vi "Channel Mng Performance Test.vi"() -> ()   [LabVIEW 2021]
uses:
  <vilib>/Platform/TimedLoop/XDataNode/XDataNode.xnode
  <vilib>/Platform/TimedLoop/XDataNode/nitl_modes.ctl
  <vilib>/Platform/TimedLoop/XDataNode/XDNodeRunTimeDep.lvlib
  <vilib>/Platform/TimedLoop/XDataNode/wakeup.ctl
  <vilib>/Platform/TimedLoop/XDataNode/timing_clust.ctl
  7d13c5b7-0b44-4ab4-8a6c-0bcd63b70b59.vi
  6a1b8880-d4c2-444f-a4b2-811244e6db06.vi
  <vilib>/CIFChannels/CIFChannelCore.lvlib
  c0ba1b46-a5a0-42bd-afb3-2f6832d2a88c.vi
  10e1b524-69ef-478e-ae98-36060d5eb0d6.vi
  332321e3-b478-4438-b8ac-43cf378b23bb.vi
  Channels/CIFTag/Double/CIFTagDouble.lvclass
  CIFChannelMng.lvclass
  D:/dev/CIF-LVCore/src/CIFUtilities/CIFChannels/CIFChannels.lvclass
panel:
  out "avg dbl channel":dbl
  out "max dbl channel":dbl
  out "avg raw channel":dbl
  out "max raw channel":dbl
  out "pass":bool
  out "error out":errorcluster
  # "This test should be run on RT.  It stresses the communications by constantly creating resource contraints with the low priority sender and the high priority loop. On Windows the priority of the loops cannot be set."
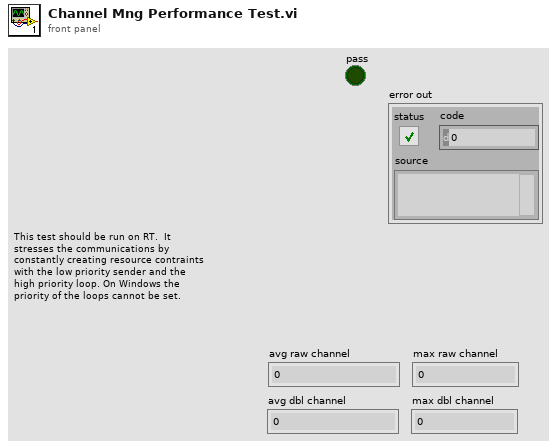
[diagram p1: front panel]
types:
  T1 = typedef "XDNodeRunTimeDep.lvlib/timing_clust.ctl" = cluster{"Expected End [f-1]":u64, "Actual End [f-1]":u64, "Finished Late? [f-1]":bool, "Expected End [i-1]":u64, "Actual End [i-1]":u64, "Finished Late? [i-1]":bool, "Expected Start [i]":u64, "Actual Start [i]":u64, "Expected Start [f]":u64, "Actual Start [f]":u64, "Source Name":string, "Structure Name":string, "Period":i64, "Deadline":i64, "Offset":i64, "Start":i64, "Priority":i32, "Timeout":i32, "Mode":T2, "Wakeup Reason":T3, "Error":errorcluster, "Source Type":string, "Secondary Source Type":string, "Global End Time":u64, "Global Start Time":u64, "Frame Duration":u64, "Iteration Duration":u64, "Assigned CPU":i32, "I/O Scan Engine Mode":u32}
  T2 = typedef "XDNodeRunTimeDep.lvlib/nitl_modes.ctl" = enum32{"No Change", "Process missed periods, maintain original phase", "Discard missed periods, maintain original phase", "Process missed periods, ignore original phase", "Discard missed periods, ignore original phase"}
  T3 = typedef "XDNodeRunTimeDep.lvlib/wakeup.ctl" = enum32{"Normal", "Aborted", "Asynchronous wakeup", "Timing source error", "Timed loop error", "Timeout"}
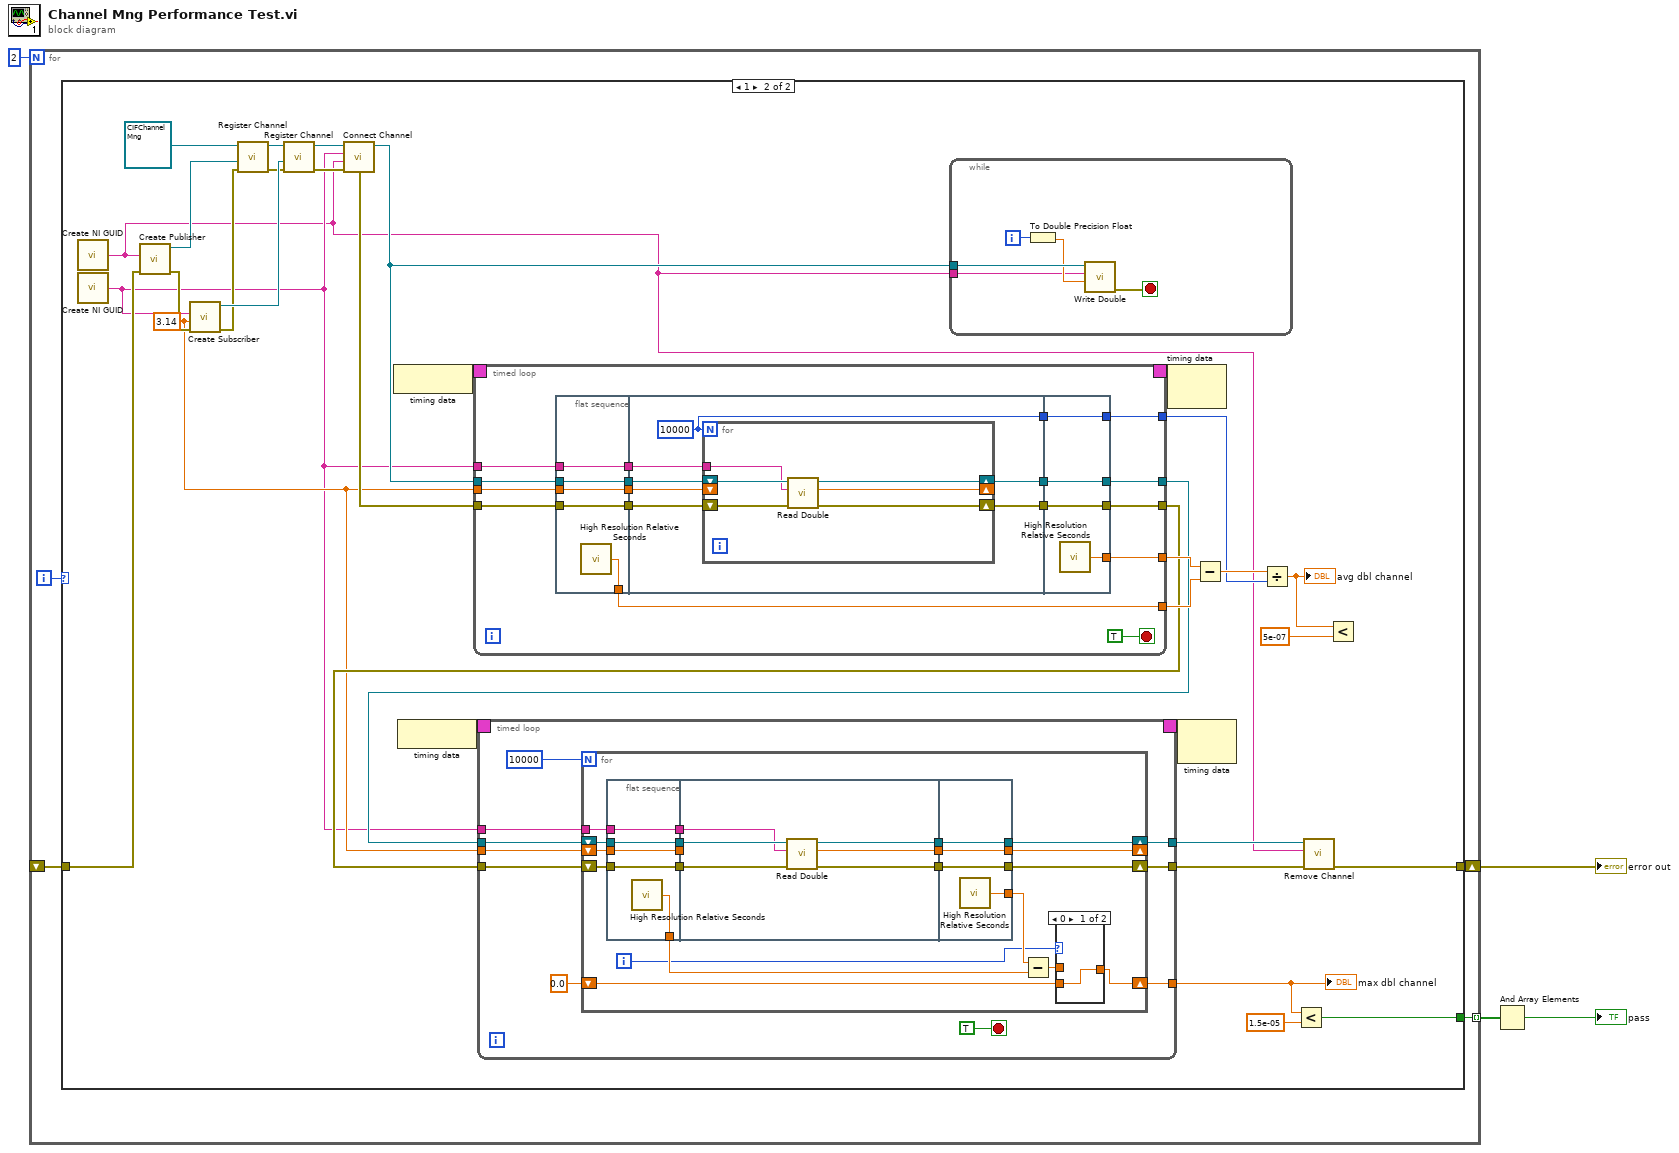
[diagram p0: block diagram]
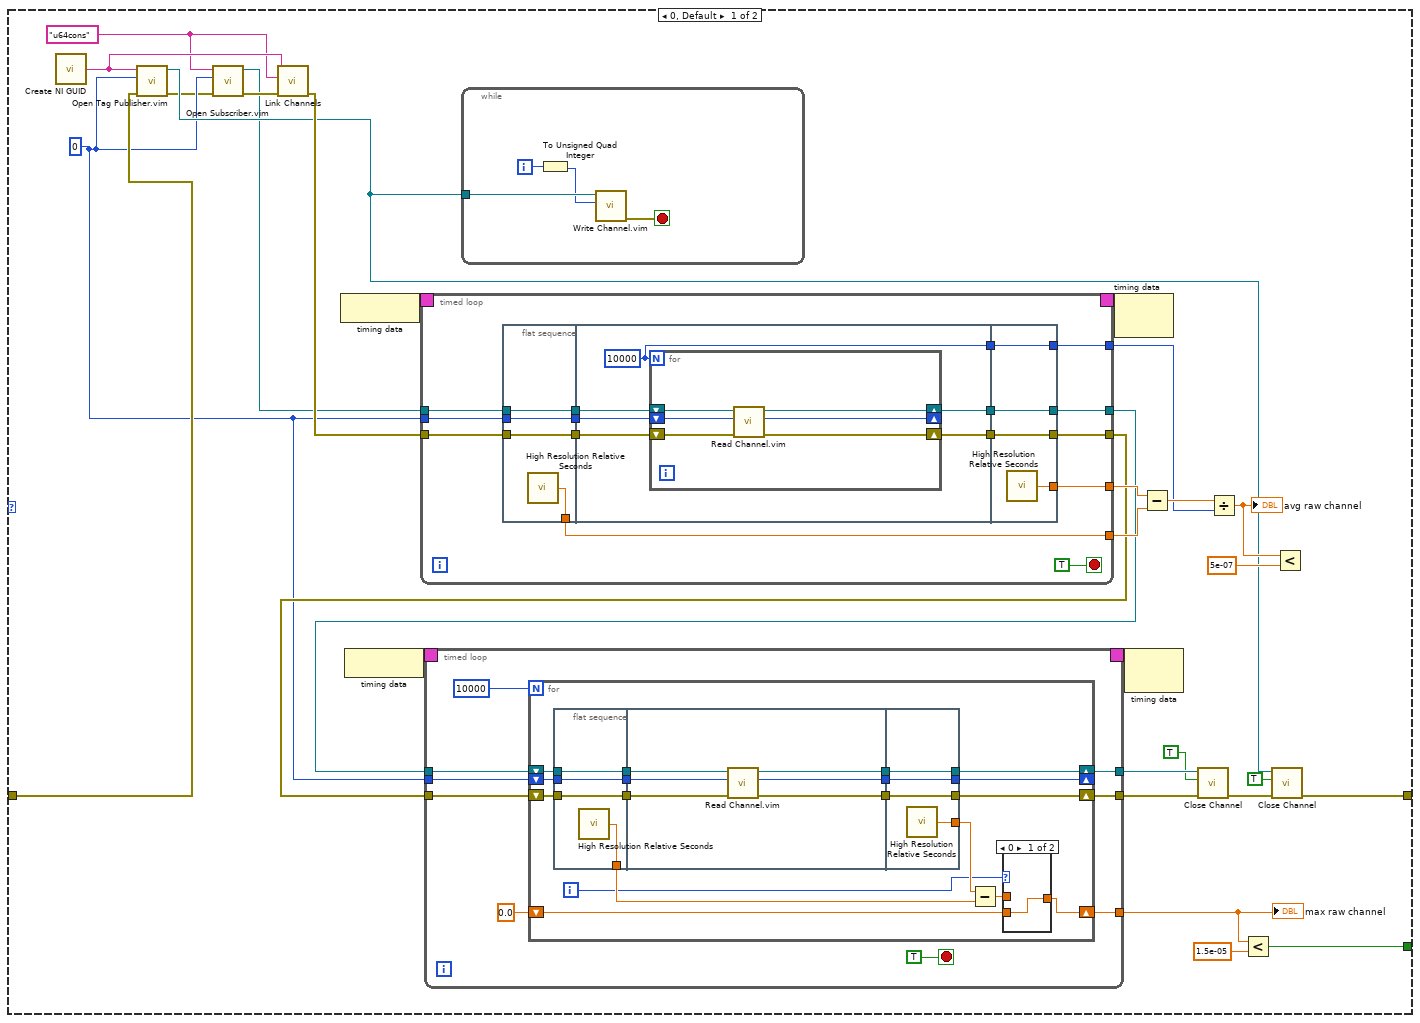
[diagram p2: hidden frame]
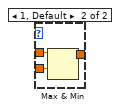
[diagram p3: hidden frame]
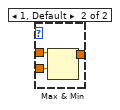
[diagram p4: hidden frame]
diagram:
  n1 = for {
    N: 2 -> [_]
    tunnel: [w8] -> w2 mode=indexing
    shift-right: [w7] -> w4
    shift-left: _ -> [w5]
    i -> [w6]
    n2 = case shown="1" w6 {
      tunnel: [w24 w149] -> w8
      tunnel: [w17 w132] -> w7
      tunnel: w5 -> [w22 w139]
      frame 0, Default {
        w11 = "u64cons" ("Channel Name")
        w13 = u64 0
        n3 = call <vilib>:"Create NI GUID.vi"() -> ("NI GUID"=w15:string)
        n4 = call "Open Tag Publisher.vim"("error in"=w22, "Input Type"=w13, "Channel Name"=w15) -> ("error out"=w12:errorcluster, "CIF Channel"=w16:refnum<k21>)  [unwired: 7 in]
        n5 = call "Open Subscriber.vim"("error in"=w12, "Input Type"=w13, "Channel Name"=w11) -> ("error out"=w10:errorcluster, "CIF Channel"=w9:refnum<k21>)  [unwired: 7 in]
        n6 = call <vilib>:"Link Channels.vi"("error in"=w10, "Consumer Channel Name"=w11, "Producer Channel Name"=w15) -> ("error out"=w23:errorcluster)  [unwired: 8 in]
        n7 = node-c288() -> (w38:T1)
        n8 = node-c288() -> (w36:T1)
        n9 = timed-loop {
          timing: w38 -> [_]
          timing-out: [_] -> w37
          tunnel: w9 -> [w106]
          tunnel: w23 -> [w105]
          tunnel: [w101] -> w30
          tunnel: [w99] -> w29
          tunnel: [w97] -> w34
          tunnel: [w96] -> w33
          tunnel: [w95] -> w31
          tunnel: w13 -> [w93]
          stop <- TRUE stop-if-true
          n10 = flat-sequence {
            tunnel: w105 -> [w109]
            tunnel: w106 -> [w110]
            tunnel: [w110] -> w103
            tunnel: [w109] -> w102
            tunnel: [w108] -> w96
            tunnel: w93 -> [w107]
            tunnel: [w107] -> w92
            tunnel: w103 -> [w116]
            tunnel: w102 -> [w115]
            tunnel: [w114] -> w100
            tunnel: [w113] -> w98
            tunnel: [w112] -> w94
            tunnel: w92 -> [w111]
            tunnel: [w126] -> w101
            tunnel: w100 -> [w126]
            tunnel: [w125] -> w99
            tunnel: w98 -> [w125]
            tunnel: [w124] -> w97
            tunnel: [w123] -> w95
            tunnel: w94 -> [w123]
            frame #0 {
              n11 = call <vilib>:"High Resolution Relative Seconds.vi"() -> ("relative seconds"=w108:dbl)
            }
            frame #1 {
              w112 = 10000
              n12 = for {
                N: w112 -> [_]
                shift-right: [w119] -> w114
                shift-left: w116 -> [w122]
                shift-right: [w118] -> w113
                shift-left: w115 -> [w117]
                shift-right: [w120] -> _
                shift-left: w111 -> [w121]
                n13 = call "Read Channel.vim"("error in"=w117, "Data in"=w121, "CIF Channel in"=w122) -> ("error out"=w118:errorcluster, "Data out"=w120:u64, "CIF Channel out"=w119:refnum<k21>)  [unwired: 5 in, 1 out]
              }
            }
            frame #2 {
              n14 = call <vilib>:"High Resolution Relative Seconds.vi"() -> ("relative seconds"=w124:dbl)
            }
          }
        }
        n15 = timed-loop {
          timing: w36 -> [_]
          timing-out: [_] -> w35
          tunnel: w30 -> [w51]
          tunnel: w29 -> [w50]
          tunnel: [w48] -> w20
          tunnel: [w47] -> w21
          tunnel: w13 -> [w46]
          tunnel: [w43] -> w26
          stop <- TRUE stop-if-true
          n16 = for {
            N: 10000 -> [_]
            shift-right: [w63] -> w48
            shift-left: w51 -> [w65]
            shift-right: [w62] -> w47
            shift-left: w50 -> [w64]
            shift-right: [w56] -> w43
            shift-left: 0.0 -> [w57]
            shift-right: [w55] -> _
            shift-left: w46 -> [w61]
            i -> [w53]
            n17 = flat-sequence {
              tunnel: w64 -> [w76]
              tunnel: w65 -> [w77]
              tunnel: [w77] -> w69
              tunnel: [w76] -> w68
              tunnel: [w75] -> w59
              tunnel: w61 -> [w74]
              tunnel: [w74] -> w67
              tunnel: w69 -> [w83]
              tunnel: w68 -> [w79]
              tunnel: [w82] -> w66
              tunnel: w67 -> [w81]
              tunnel: [w80] -> w54
              tunnel: [w78] -> w52
              tunnel: [w87] -> w63
              tunnel: w66 -> [w87]
              tunnel: [w86] -> w62
              tunnel: [w85] -> w60
              tunnel: [w84] -> w55
              tunnel: w54 -> [w84]
              tunnel: w52 -> [w86]
              frame #0 {
                n18 = call <vilib>:"High Resolution Relative Seconds.vi"() -> ("relative seconds"=w75:dbl)
              }
              frame #1 {
                n19 = call "Read Channel.vim"("error in"=w79, "Data in"=w81, "CIF Channel in"=w83) -> ("error out"=w78:errorcluster, "Data out"=w80:u64, "CIF Channel out"=w82:refnum<k21>)  [unwired: 5 in, 1 out]
              }
              frame #2 {
                n20 = call <vilib>:"High Resolution Relative Seconds.vi"() -> ("relative seconds"=w85:dbl)
              }
            }
            n21 = Subtract(x=w60, y=w59) -> (x-y=w58:dbl)
            n22 = case shown="0" w53 {
              tunnel: w58 -> [_ w73]
              tunnel: w57 -> [w70 w72]
              tunnel: [w70 w71] -> w56
              frame 0 {
              }
              frame 1, Default {
                n23 = Max & Min(x=w73, y=w72) -> (max(x,y)=w71:dbl)  [unwired: 1 out]
              }
            }
          }
        }
        "max raw channel" <- w26
        n24 = while {
          tunnel: w16 -> [w41]
          i -> [w42]
          stop <- w39 stop-if-true
          n25 = To Unsigned Quad Integer(1:w42) -> (0:w40:u64)
          n26 = call "Write Channel.vim"("Data in"=w40, "CIF Channel in"=w41) -> ("error out"=w39:errorcluster)  [unwired: 6 in, 3 out]
        }
        n27 = node-c288(w37) -> ()  [unwired: 1 out]
        n28 = node-c288(w35) -> ()  [unwired: 1 out]
        n29 = Subtract(x=w34, y=w33) -> (x-y=w32:dbl)
        n30 = call <vilib>:"Close Channel.vi"("error in"=w21, "Force Destroy? (F)"=TRUE, "CIF Channel"=w20) -> ("error out"=w19:errorcluster)  [unwired: 8 in]
        n31 = Divide(x=w32, y=w31) -> (x/y=w28:dbl)
        "avg raw channel" <- w28
        n32 = Less?(x=w26, y=1.5e-05) -> (x < y?=w24:bool)
        n33 = call <vilib>:"Close Channel.vi"("error in"=w19, "Force Destroy? (F)"=TRUE, "CIF Channel"=w16) -> ("error out"=w17:errorcluster)  [unwired: 8 in]
        n34 = Less?(x=w28, y=5e-07) -> ()  [unwired: 1 out]
      }
      frame 1 {
        w136 = 3.14 ("Default Value")
        n35 = call <vilib>:"Create NI GUID.vi"() -> ("NI GUID"=w131:string)
        n36 = call <vilib>:"Create NI GUID.vi"() -> ("NI GUID"=w135:string)
        n37 = call "Create Publisher.vi"("error in (no error)"=w139, "Name"=w131) -> ("error out"=w144:errorcluster, "CIFTag out"=w143:refnum<class "CIFTagDouble.lvclass">)  [unwired: 8 in]
        n38 = call "Create Subscriber.vi"("error in (no error)"=w144, "Default Value"=w136, "Name"=w135) -> ("error out"=w145:errorcluster, "CIFTag out"=w148:refnum<class "CIFTagDouble.lvclass">)  [unwired: 7 in]
        n39 = call "Register Channel.vi"("error in (no error)"=w145, "Channel"=w143, "CIFChannelMng in"=refnum<class "CIFChannelMng.lvclass"> refnum) -> ("error out"=w142:errorcluster, "CIFChannelMng out"=w141:refnum<class "CIFChannelMng.lvclass">)  [unwired: 7 in]
        n40 = call "Register Channel.vi"("error in (no error)"=w142, "Channel"=w148, "CIFChannelMng in"=w141) -> ("error out"=w147:errorcluster, "CIFChannelMng out"=w146:refnum<class "CIFChannelMng.lvclass">)  [unwired: 7 in]
        n41 = call "Connect Channel.vi"("error in (no error)"=w147, "Publisher Name"=w131, "Subscriber Name"=w135, "CIFChannelMng in"=w146) -> ("error out"=w138:errorcluster, "CIFChannelMng out"=w137:refnum<class "CIFChannelMng.lvclass">)  [unwired: 6 in]
        n42 = node-c288() -> (w163:T1)
        n43 = node-c288() -> (w161:T1)
        n44 = timed-loop {
          timing: w163 -> [_]
          timing-out: [_] -> w162
          tunnel: w137 -> [w238]
          tunnel: w138 -> [w237]
          tunnel: [w233] -> w155
          tunnel: [w231] -> w154
          tunnel: [w229] -> w159
          tunnel: [w228] -> w158
          tunnel: [w227] -> w156
          tunnel: w136 -> [w225]
          tunnel: w135 -> [w223]
          stop <- TRUE stop-if-true
          n45 = flat-sequence {
            tunnel: w237 -> [w242]
            tunnel: w238 -> [w243]
            tunnel: [w243] -> w235
            tunnel: [w242] -> w234
            tunnel: [w241] -> w228
            tunnel: w225 -> [w240]
            tunnel: [w240] -> w224
            tunnel: w223 -> [w239]
            tunnel: [w239] -> w222
            tunnel: w235 -> [w250]
            tunnel: w234 -> [w249]
            tunnel: [w248] -> w232
            tunnel: [w247] -> w230
            tunnel: [w246] -> w226
            tunnel: w224 -> [w245]
            tunnel: w222 -> [w244]
            tunnel: [w260] -> w233
            tunnel: w232 -> [w260]
            tunnel: [w259] -> w231
            tunnel: w230 -> [w259]
            tunnel: [w258] -> w229
            tunnel: [w257] -> w227
            tunnel: w226 -> [w257]
            frame #0 {
              n46 = call <vilib>:"High Resolution Relative Seconds.vi"() -> ("relative seconds"=w241:dbl)
            }
            frame #1 {
              w246 = 10000
              n47 = for {
                N: w246 -> [_]
                shift-right: [w255] -> w248
                shift-left: w250 -> [w256]
                shift-right: [w254] -> w247
                shift-left: w249 -> [w253]
                shift-right: [w252] -> _
                shift-left: w245 -> [_]
                tunnel: w244 -> [w251]
                n48 = call "Read Double.vi"("error in (no error)"=w253, "Channel Name"=w251, "CIFChannelMng in"=w256) -> ("error out"=w254:errorcluster, "Data"=w252:dbl, "CIFChannelMng out"=w255:refnum<class "CIFChannelMng.lvclass">)  [unwired: 5 in, 1 out]
              }
            }
            frame #2 {
              n49 = call <vilib>:"High Resolution Relative Seconds.vi"() -> ("relative seconds"=w258:dbl)
            }
          }
        }
        n50 = timed-loop {
          timing: w161 -> [_]
          timing-out: [_] -> w160
          tunnel: w155 -> [w178]
          tunnel: w154 -> [w177]
          tunnel: [w175] -> w134
          tunnel: [w174] -> w133
          tunnel: w136 -> [w173]
          tunnel: [w170] -> w151
          tunnel: w135 -> [w169]
          stop <- TRUE stop-if-true
          n51 = for {
            N: 10000 -> [_]
            shift-right: [w192] -> w175
            shift-left: w178 -> [w194]
            shift-right: [w191] -> w174
            shift-left: w177 -> [w193]
            shift-right: [w185] -> w170
            shift-left: 0.0 -> [w186]
            shift-right: [w184] -> _
            shift-left: w173 -> [w190]
            tunnel: w169 -> [w180]
            i -> [w182]
            n52 = flat-sequence {
              tunnel: w193 -> [w206]
              tunnel: w194 -> [w207]
              tunnel: [w207] -> w198
              tunnel: [w206] -> w197
              tunnel: [w205] -> w188
              tunnel: w190 -> [w204]
              tunnel: [w204] -> w196
              tunnel: w180 -> [w203]
              tunnel: [w203] -> w179
              tunnel: w198 -> [w212]
              tunnel: w197 -> [w213]
              tunnel: [w211] -> w195
              tunnel: w196 -> [_]
              tunnel: [w209] -> w183
              tunnel: [w210] -> w181
              tunnel: w179 -> [w208]
              tunnel: [w217] -> w192
              tunnel: w195 -> [w217]
              tunnel: [w216] -> w191
              tunnel: [w215] -> w189
              tunnel: [w214] -> w184
              tunnel: w183 -> [w214]
              tunnel: w181 -> [w216]
              frame #0 {
                n53 = call <vilib>:"High Resolution Relative Seconds.vi"() -> ("relative seconds"=w205:dbl)
              }
              frame #1 {
                n54 = call "Read Double.vi"("error in (no error)"=w213, "Channel Name"=w208, "CIFChannelMng in"=w212) -> ("error out"=w210:errorcluster, "Data"=w209:dbl, "CIFChannelMng out"=w211:refnum<class "CIFChannelMng.lvclass">)  [unwired: 5 in, 1 out]
              }
              frame #2 {
                n55 = call <vilib>:"High Resolution Relative Seconds.vi"() -> ("relative seconds"=w215:dbl)
              }
            }
            n56 = Subtract(x=w189, y=w188) -> (x-y=w187:dbl)
            n57 = case shown="0" w182 {
              tunnel: w187 -> [_ w202]
              tunnel: w186 -> [w199 w201]
              tunnel: [w199 w200] -> w185
              frame 0 {
              }
              frame 1, Default {
                n58 = Max & Min(x=w202, y=w201) -> (max(x,y)=w200:dbl)  [unwired: 1 out]
              }
            }
          }
        }
        "max dbl channel" <- w151
        n59 = while {
          tunnel: w137 -> [w167]
          tunnel: w131 -> [w164]
          i -> [w168]
          stop <- w165 stop-if-true
          n60 = To Double Precision Float(number=w168) -> (double precision float=w166:dbl)
          n61 = call "Write Double.vi"("Data"=w166, "Channel Name"=w164, "CIFChannelMng in"=w167) -> ("error out"=w165:errorcluster)  [unwired: 6 in, 2 out]
        }
        n62 = node-c288(w162) -> ()  [unwired: 1 out]
        n63 = node-c288(w160) -> ()  [unwired: 1 out]
        n64 = Subtract(x=w159, y=w158) -> (x-y=w157:dbl)
        n65 = Divide(x=w157, y=w156) -> (x/y=w153:dbl)
        "avg dbl channel" <- w153
        n66 = Less?(x=w151, y=1.5e-05) -> (x < y?=w149:bool)
        n67 = call "Remove Channel.vi"("error in (no error)"=w133, "Channel Name"=w131, "CIFChannelMng in"=w134) -> ("error out"=w132:errorcluster)  [unwired: 7 in, 1 out]
        n68 = Less?(x=w153, y=5e-07) -> ()  [unwired: 1 out]
      }
    }
  }
  "error out" <- w4
  n69 = And Array Elements(Boolean array=w2) -> (logical AND=→"pass":bool)
